vi "readForceSensor.vi"(8 "error in (no error)":errorcluster, 11 "Bootloader in":refnum<class "Bootloader.lvclass">) -> (0 "error out":errorcluster, 2 "Force Sensor Settings":T1={"ADC Channel"=1, "Reference Voltage Vref"=0.0} {"Reference Voltage Vref" min=-10.0 max=10.0 format="%.3f"}, 3 "Bootloader out":refnum<class "Bootloader.lvclass">)   [LabVIEW 2015, in "Bootloader.lvclass"]
uses:
  Bootloader.lvclass
  Typedefs/ForceSensorSettings.ctl
  ConfigurationTestParameters/ConfigurationTestParameters.lvclass
  Typedefs/FAMTTypedefs.lvlib
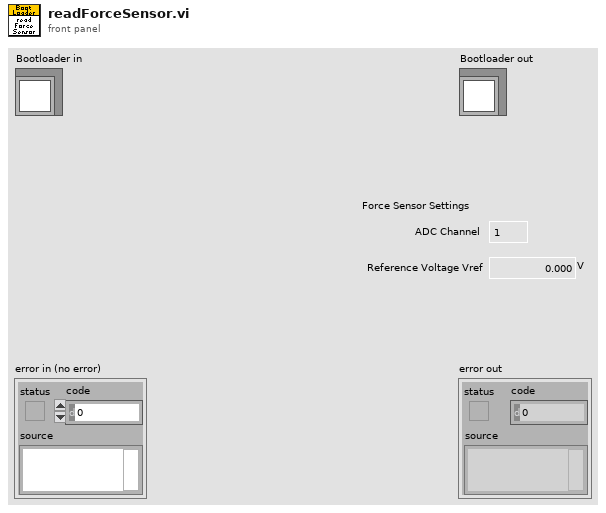
[diagram p1: front panel]
types:
  T1 = typedef "FAMTTypedefs.lvlib/ForceSensorSettings.ctl" = cluster{"ADC Channel":u8, "Reference Voltage Vref":dbl[unit]}
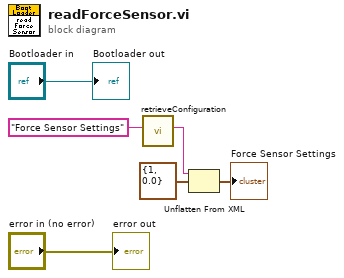
[diagram p0: block diagram]
diagram:
  n1 = call "retrieveConfiguration.vi"("configName"="Force Sensor Settings") -> ("xmlConfig"=w3:string)  [unwired: 8 in, 2 out]
  n2 = Unflatten From XML(xml string=w3, type=T1 {"ADC Channel"=1, "Reference Voltage Vref"=0.0} ("Force Sensor Settings")) -> (value=→"Force Sensor Settings":T1)  [unwired: 1 in, 1 out]
  "error out" <- "error in (no error)"
  "Bootloader out" <- "Bootloader in"
